vi "SearchandUpdateValues.vi"(10 "Contents":string[](array[string]), 11 "Rules":string[][](array[string])) -> (3 "New Contents":string[](array[string]))   [LabVIEW 2015, in "ReportList.lvclass"]
uses:
  ReportList.lvclass
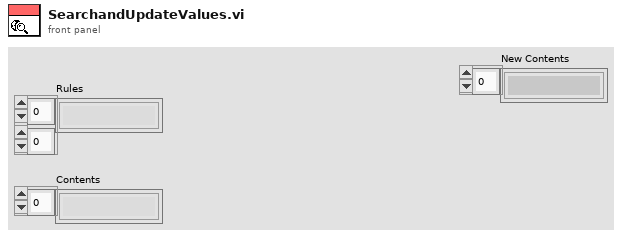
[diagram p1: front panel]
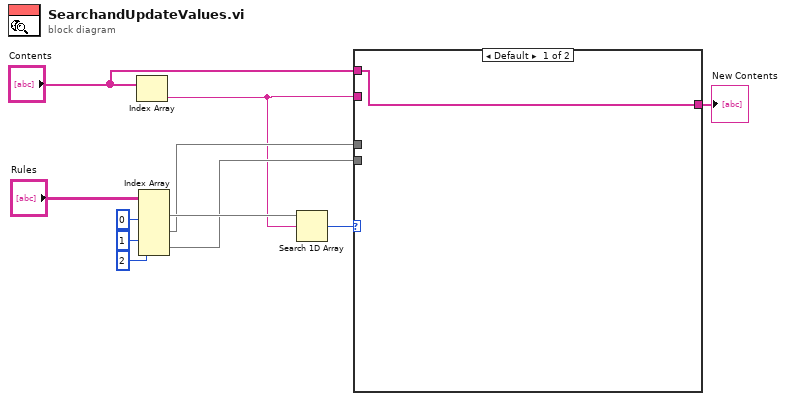
[diagram p0: block diagram]
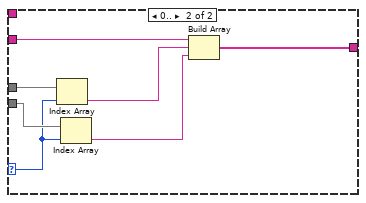
[diagram p2: hidden frame]
diagram:
  n1 = Index Array(array="Contents") -> (element=w3:string)  [unwired: 1 in]
  n2 = Index Array(array="Rules", index (col) #1=0 ("disabled index (col)"), index (col) #2=1 ("index (col)"), index (col) #3=2 ("index (col)")) -> (element #1=w7:string[], element #2=w5:string[], element #3=w4:string[])  [unwired: 3 in]
  n3 = Search 1D Array(1D array=w7, element=w3) -> (index of element=w6:i32)  [unwired: 1 in]
  n4 = case shown="Default" w6 {
    selector: w6 -> [_ w17]
    tunnel: w5 -> [_ w19]
    tunnel: w4 -> [_ w18]
    tunnel: w3 -> [_ w16]
    tunnel: [w12 w13] -> w2
    tunnel: "Contents" -> [w12 _]
    frame Default {
    }
    frame 0.. {
      n5 = Index Array(array=w19, index=w17) -> (element=w15:string)
      n6 = Index Array(array=w18, index=w17) -> (element=w14:string)
      n7 = Build Array(w16, w15, w14) -> (w13:string[])
    }
  }
  "New Contents" <- w2
